vi "CompileMaster_Old.vi"(4 "Compiler Settings":T1={"Python Path"=path "", "Main File"="makesequence.py", "Meta File"="makesequence.py", "Aux File"="C:\\Python27"}, 6 "step num":i32, 7 "Master Exp In":T2) -> (0 "Standard Error Out":string, 2 "Experiment Text":string, 3 "Master Exp Out":T2)   [LabVIEW 2017]
uses:
  controls/MasterExperiment.ctl
  PulseCompiler/CompilerSettings.ctl
  PulseCompiler/SequenceCluster.ctl
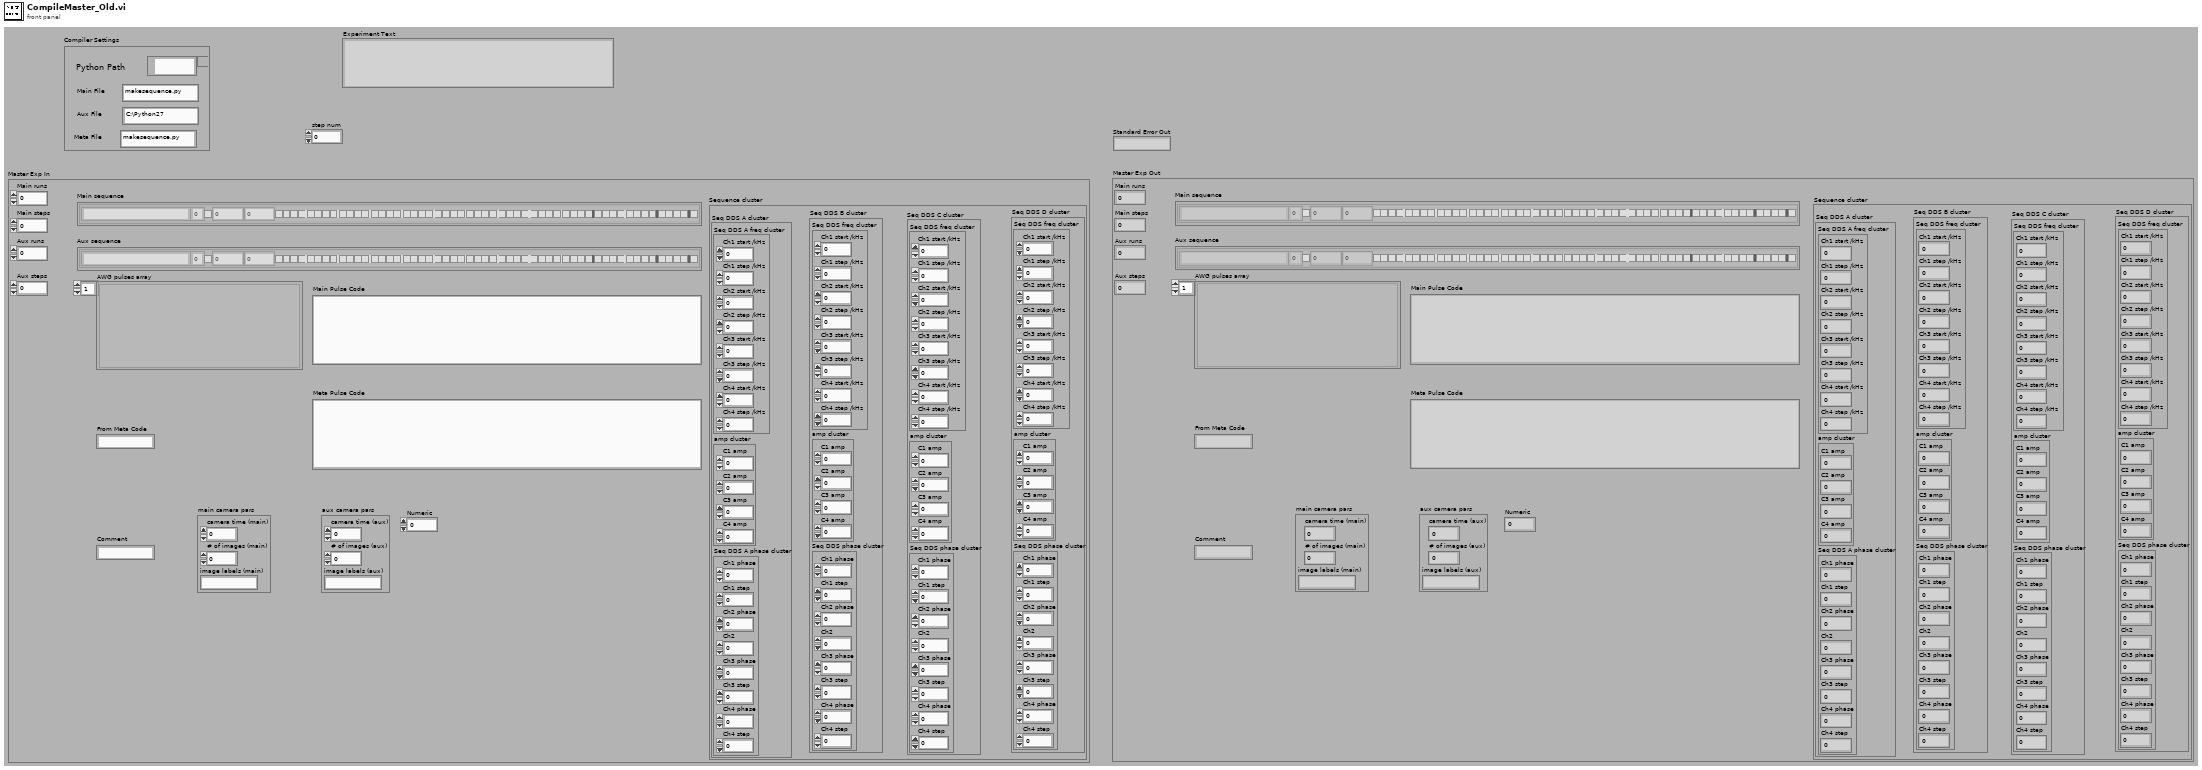
[diagram p1: front panel]
types:
  T1 = typedef "CompilerSettings.ctl" = cluster{"Python Path":path, "Main File":string, "Meta File":string, "Aux File":string}
  T2 = typedef "MasterExperiment.ctl" = cluster{"Main runs":dbl, "Numeric":dbl, "Main steps":dbl, "Aux runs":dbl, "Aux steps":dbl, "Main sequence":cluster{"Pulse name":string, "Pulse number":i32, "Enabled?":bool, "Time":dbl, "Step":dbl, "Pulse 0":bool, "Pulse 1":bool, "Pulse 2":bool, "Pulse 3":bool, "Pulse 4":bool, "Pulse 5":bool, "Pulse 6":bool, "Pulse 7":bool, "Pulse 8":bool, "Pulse 9":bool, "Pulse 10":bool, "Pulse 11":bool, "Pulse 12":bool, "Pulse 13":bool, "Pulse 14":bool, "Pulse 15":bool, "Pulse 16":bool, "Pulse 17":bool, "Pulse 18":bool, "Pulse 19":bool, "Pulse 20":bool, "Pulse 21":bool, "Pulse 22":bool, "Pulse 23":bool, "Pulse 24":bool, "Pulse 25":bool, "Pulse 26":bool, "Pulse 27":bool, "Pulse 28":bool, "Pulse 29":bool, "Pulse 30":bool, "Pulse 31":bool, "Pulse 32":bool, "Pulse 33":bool, "Pulse 34":bool, "Pulse 35":bool, "Pulse 36":bool, "Pulse 37":bool, "Pulse 38":bool, "Pulse 39":bool, "Count 0":bool, "Count 1":bool, "Count 2":bool, "Count 3":bool, "Count 4":bool, "Count 5":bool, "Count 6":bool, "Count 7":bool, "AO 0":bool, "AO 1":bool, "AO 2":bool, "AO 3":bool, "Trigger 0":bool}[], "Aux sequence":cluster{"Pulse name":string, "Pulse number":i32, "Enabled?":bool, "Time":dbl, "Step":dbl, "Pulse 0":bool, "Pulse 1":bool, "Pulse 2":bool, "Pulse 3":bool, "Pulse 4":bool, "Pulse 5":bool, "Pulse 6":bool, "Pulse 7":bool, "Pulse 8":bool, "Pulse 9":bool, "Pulse 10":bool, "Pulse 11":bool, "Pulse 12":bool, "Pulse 13":bool, "Pulse 14":bool, "Pulse 15":bool, "Pulse 16":bool, "Pulse 17":bool, "Pulse 18":bool, "Pulse 19":bool, "Pulse 20":bool, "Pulse 21":bool, "Pulse 22":bool, "Pulse 23":bool, "Pulse 24":bool, "Pulse 25":bool, "Pulse 26":bool, "Pulse 27":bool, "Pulse 28":bool, "Pulse 29":bool, "Pulse 30":bool, "Pulse 31":bool, "Pulse 32":bool, "Pulse 33":bool, "Pulse 34":bool, "Pulse 35":bool, "Pulse 36":bool, "Pulse 37":bool, "Pulse 38":bool, "Pulse 39":bool, "Count 0":bool, "Count 1":bool, "Count 2":bool, "Count 3":bool, "Count 4":bool, "Count 5":bool, "Count 6":bool, "Count 7":bool, "AO 0":bool, "AO 1":bool, "AO 2":bool, "AO 3":bool, "Trigger 0":bool}[], "AWG pulses array":variant[], "Main Pulse Code":string, "Meta Pulse Code":string, "Comment":string, "main camera pars":cluster{"camera time (main)":i32, "# of images (main)":i32, "image labels (main)":string}, "aux camera pars":cluster{"camera time (aux)":i32, "# of images (aux)":i32, "image labels (aux)":string}, "From Meta Code":string, "Sequence cluster":T3}
  T3 = typedef "SequenceCluster.ctl" = cluster{"Seq DDS A cluster":cluster{"Seq DDS A freq cluster":cluster{"Ch1 start /kHz":dbl, "Ch1 step /kHz":dbl, "Ch2 start /kHz":dbl, "Ch2 step /kHz":dbl, "Ch3 start /kHz":dbl, "Ch3 step /kHz":dbl, "Ch4 start /kHz":dbl, "Ch4 step /kHz":dbl}, "amp cluster":cluster{"C1 amp":dbl, "C2 amp":dbl, "C3 amp":dbl, "C4 amp":dbl}, "Seq DDS A phase cluster":cluster{"Ch1 phase":dbl, "Ch1 step":dbl, "Ch2 phase":dbl, "Ch2":dbl, "Ch3 phase":dbl, "Ch3 step":dbl, "Ch4 phase":dbl, "Ch4 step":dbl}}, "Seq DDS B cluster":cluster{"Seq DDS freq cluster":cluster{"Ch1 start /kHz":dbl, "Ch1 step /kHz":dbl, "Ch2 start /kHz":dbl, "Ch2 step /kHz":dbl, "Ch3 start /kHz":dbl, "Ch3 step /kHz":dbl, "Ch4 start /kHz":dbl, "Ch4 step /kHz":dbl}, "amp cluster":cluster{"C1 amp":dbl, "C2 amp":dbl, "C3 amp":dbl, "C4 amp":dbl}, "Seq DDS phase cluster":cluster{"Ch1 phase":dbl, "Ch1 step":dbl, "Ch2 phase":dbl, "Ch2":dbl, "Ch3 phase":dbl, "Ch3 step":dbl, "Ch4 phase":dbl, "Ch4 step":dbl}}, "Seq DDS C cluster":cluster{"Seq DDS freq cluster":cluster{"Ch1 start /kHz":dbl, "Ch1 step /kHz":dbl, "Ch2 start /kHz":dbl, "Ch2 step /kHz":dbl, "Ch3 start /kHz":dbl, "Ch3 step /kHz":dbl, "Ch4 start /kHz":dbl, "Ch4 step /kHz":dbl}, "amp cluster":cluster{"C1 amp":dbl, "C2 amp":dbl, "C3 amp":dbl, "C4 amp":dbl}, "Seq DDS phase cluster":cluster{"Ch1 phase":dbl, "Ch1 step":dbl, "Ch2 phase":dbl, "Ch2":dbl, "Ch3 phase":dbl, "Ch3 step":dbl, "Ch4 phase":dbl, "Ch4 step":dbl}}, "Seq DDS D cluster":cluster{"Seq DDS freq cluster":cluster{"Ch1 start /kHz":dbl, "Ch1 step /kHz":dbl, "Ch2 start /kHz":dbl, "Ch2 step /kHz":dbl, "Ch3 start /kHz":dbl, "Ch3 step /kHz":dbl, "Ch4 start /kHz":dbl, "Ch4 step /kHz":dbl}, "amp cluster":cluster{"C1 amp":dbl, "C2 amp":dbl, "C3 amp":dbl, "C4 amp":dbl}, "Seq DDS phase cluster":cluster{"Ch1 phase":dbl, "Ch1 step":dbl, "Ch2 phase":dbl, "Ch2":dbl, "Ch3 phase":dbl, "Ch3 step":dbl, "Ch4 phase":dbl, "Ch4 step":dbl}}}
  T4 = cluster{"Main sequence":string, "Aux sequence":string, "Camera":string, "RF":string, "Pars":string, "Synths":string}
  T5 = cluster{"Main runs":dbl, "Main steps":dbl, "Comment":string}
  T6 = cluster{"# of runs":i32, "# of steps":i32, "comment":string}
  T7 = cluster{"Pulse name":string, "Pulse number":i32, "Enabled?":bool, "Time":dbl, "Step":dbl, "Pulse 0":bool, "Pulse 1":bool, "Pulse 2":bool, "Pulse 3":bool, "Pulse 4":bool, "Pulse 5":bool, "Pulse 6":bool, "Pulse 7":bool, "Pulse 8":bool, "Pulse 9":bool, "Pulse 10":bool, "Pulse 11":bool, "Pulse 12":bool, "Pulse 13":bool, "Pulse 14":bool, "Pulse 15":bool, "Pulse 16":bool, "Pulse 17":bool, "Pulse 18":bool, "Pulse 19":bool, "Pulse 20":bool, "Pulse 21":bool, "Pulse 22":bool, "Pulse 23":bool, "Pulse 24":bool, "Pulse 25":bool, "Pulse 26":bool, "Pulse 27":bool, "Pulse 28":bool, "Pulse 29":bool, "Pulse 30":bool, "Pulse 31":bool, "Pulse 32":bool, "Pulse 33":bool, "Pulse 34":bool, "Pulse 35":bool, "Pulse 36":bool, "Pulse 37":bool, "Pulse 38":bool, "Pulse 39":bool, "Count 0":bool, "Count 1":bool, "Count 2":bool, "Count 3":bool, "Count 4":bool, "Count 5":bool, "Count 6":bool, "Count 7":bool, "AO 0":bool, "AO 1":bool, "AO 2":bool, "AO 3":bool, "Trigger 0":bool}[]
  T8 = cluster{"camera time (aux)":i32, "# of images (aux)":i32, "image labels (aux)":string}
  T9 = cluster{"camera time (main)":i32, "# of images (main)":i32, "image labels (main)":string}
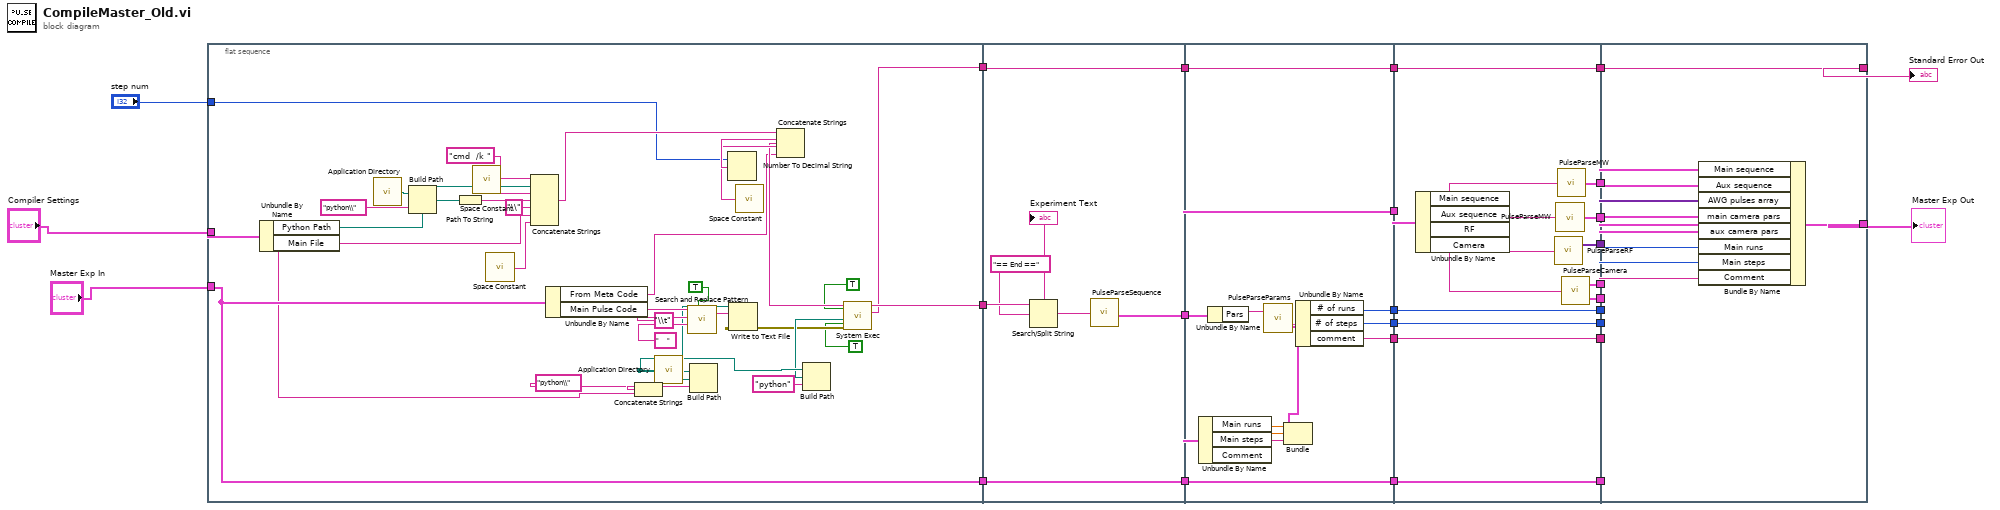
[diagram p0: block diagram]
diagram:
  n1 = flat-sequence {
    tunnel: "Master Exp In" -> [w45]
    tunnel: [w46] -> w26
    tunnel: [w45] -> w24
    tunnel: [w44] -> w7
    tunnel: "Compiler Settings" -> [w41]
    tunnel: "step num" -> [w29]
    tunnel: w26 -> [w67]
    tunnel: [w64] -> w25
    tunnel: w24 -> [w64]
    tunnel: [w63] -> w23
    tunnel: [w62] -> w8
    tunnel: w7 -> [w62]
    tunnel: w25 -> [w73]
    tunnel: w23 -> [w74]
    tunnel: [w74] -> w22
    tunnel: [w73] -> w20
    tunnel: [w71] -> w13
    tunnel: [w70] -> w11
    tunnel: [w69] -> w9
    tunnel: w8 -> [w69]
    tunnel: [w68] -> w4
    tunnel: w22 -> [w94]
    tunnel: [w89] -> w21
    tunnel: w20 -> [w89]
    tunnel: [w88] -> w19
    tunnel: [w87] -> w18
    tunnel: [w86] -> w17
    tunnel: [w85] -> w16
    tunnel: [w84] -> w15
    tunnel: [w83] -> w14
    tunnel: w13 -> [w83]
    tunnel: [w82] -> w12
    tunnel: w11 -> [w82]
    tunnel: [w81] -> w10
    tunnel: w9 -> [w81]
    tunnel: [w80] -> w5
    tunnel: w4 -> [w80]
    tunnel: w21 -> [w105]
    tunnel: w19 -> [w104]
    tunnel: w18 -> [w103]
    tunnel: w17 -> [w102]
    tunnel: w16 -> [w101]
    tunnel: w15 -> [w100]
    tunnel: w14 -> [w99]
    tunnel: w12 -> [w98]
    tunnel: w10 -> [w97]
    tunnel: [w97] -> w6
    tunnel: w5 -> [w96]
    tunnel: [w95] -> w3
    frame #0 {
      n2 = Unbundle By Name(w41) -> ("Python Path"=w39:path, "Main File"=w32:string)
      n3 = call <vilib>:"Application Directory.vi"() -> ("Application Directory"=w36:path)
      n4 = Build Path(base path=w36, name or relative path="python\\") -> (appended path=w34:path)
      n5 = Path To String(path=w34) -> (string=w33:string)
      n6 = call <vilib>:"Space Constant.vi"() -> ("String"=w38:string)
      n7 = call <vilib>:"Space Constant.vi"() -> ("String"=w31:string)
      n8 = Concatenate Strings("cmd  /k " ("string"), w39, w38, w33, "\\" ("string"), w32, w31) -> (w37:string)
      n9 = Unbundle By Name(w45) -> ("From Meta Code"=w28:string, "Main Pulse Code"=w58:string)
      n10 = Concatenate Strings("python\\" ("name or relative path"), w32) -> (w43:string)
      n11 = call <vilib>:"Application Directory.vi"() -> ("Application Directory"=w52:path)
      n12 = call <vilib>:"Search and Replace Pattern.vi"("string"=w58, "regular expression (\"\")"="\\t" ("regular expression (\"\")"), "replace string (\"\")"="    " ("replace string (\"\")"), "replace all? (F)"=TRUE) -> ("result string"=w57:string)  [unwired: 1 in, 1 out]
      n13 = Build Path(base path=w52, name or relative path=w43) -> (appended path=w56:path)
      n14 = Number To Decimal String(number=w29) -> (decimal integer string=w55:string)  [unwired: 1 in]
      n15 = Write to Text File(file (use dialog)=w56, text=w57) -> (error out=w49:errorcluster)  [unwired: 2 in, 2 out]
      n16 = call <vilib>:"Space Constant.vi"() -> ("String"=w54:string)
      n17 = Concatenate Strings(w37, w55, w54, w28) -> (w53:string)
      n18 = Build Path(base path=w52, name or relative path="python") -> (appended path=w50:path)
      n19 = call <vilib>:"System Exec.vi"("run minimized? (F)"=TRUE, "wait until completion? (T)"=TRUE, "error in (no error)"=w49, "working directory"=w50, "command line"=w53) -> ("standard error"=w44:string, "standard output"=w46:string)  [unwired: 3 in, 2 out]
    }
    frame #1 {
      n20 = Search/Split String(string=w67, search string/char (-)="== End ==") -> (substring before match=w65:string)  [unwired: 1 in, 2 out]
      "Experiment Text" <- w65
      n21 = call "PulseParseSequence.vi"("String"=w65) -> ("pulses cluster"=w63:T4)  [unwired: 1 out]
    }
    frame #2 {
      n22 = Unbundle By Name(w73) -> ("Main runs"=w79:dbl, "Main steps"=w78:dbl, "Comment"=w77:string)
      n23 = Unbundle By Name(w74) -> ("Pars"=w75:string)
      n24 = Bundle("Main runs"=w79, "Main steps"=w78, "Comment"=w77) -> (w76:T5)  [unwired: 1 in]
      n25 = call "PulseParseParams.vi"("Pars cluster"=w76, "Pars String"=w75) -> ("Pars cluster"=w72:T6)  [unwired: 1 out]
      n26 = Unbundle By Name(w72) -> ("# of runs"=w71:i32, "# of steps"=w70:i32, "comment"=w68:string)
    }
    frame #3 {
      n27 = Unbundle By Name(w94) -> ("Main sequence"=w92:string, "Aux sequence"=w91:string, "RF"=w93:string, "Camera"=w90:string)
      n28 = call "PulseParseRF.vi"("String"=w93) -> ("Array"=w86:variant[])  [unwired: 1 in]
      n29 = call "PulseParseMW.vi"("String"=w91) -> ("Full Pulse Array"=w87:T7)
      n30 = call "PulseParseMW.vi"("String"=w92) -> ("Full Pulse Array"=w88:T7)
      n31 = call "PulseParseCamera.vi"("Pars String"=w90) -> ("aux camera pars"=w84:T8, "main camera pars"=w85:T9)
    }
    frame #4 {
      n32 = Bundle By Name(cluster=w105, "Main sequence"=w104, "Aux sequence"=w103, "AWG pulses array"=w102, "main camera pars"=w101, "aux camera pars"=w100, "Main runs"=w99, "Main steps"=w98, "Comment"=w96) -> (w95:T2)
    }
  }
  "Standard Error Out" <- w6
  "Master Exp Out" <- w3
